vi "InitializeCamera.vi"() -> ()   [LabVIEW 2015]
uses:
  MVCAMSDK.dll
panel:
  in  "相机枚举":T1(ring)
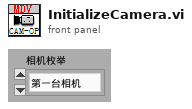
[diagram p1: front panel]
types:
  T1 = enum16{"第一台相机", "第二台相机", "第三台相机", "第四台相机", "第五台相机"}
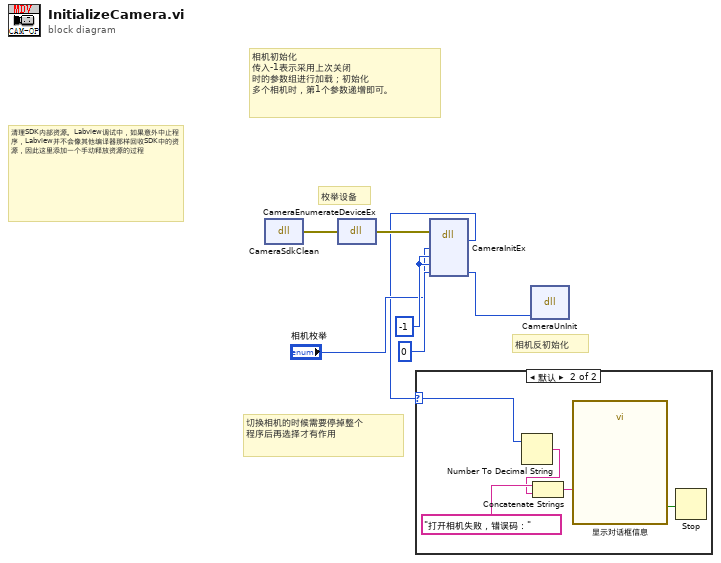
[diagram p0: block diagram]
diagram:
  w6 = -1
  # "相机反初始化"
  # "切换相机的时候需要停掉整个\n程序后再选择才有作用"
  # "清理SDK内部资源。Labview调试中，如果意外中止程序，Labview并不会像其他编译器那样回收SDK中的资源，因此这里添加一个手动释放资源的过程"
  # "相机初始化\n传入-1表示采用上次关闭\n时的参数组进行加载；初始化\n多个相机时，第1个参数递增即可。"
  # "枚举设备"
  n1 = dll-call lib="MVCAMSDK.dll" fn="CameraSdkClean"() -> (error out=w7:errorcluster)  [unwired: 4 in, 1 out]
  n2 = dll-call lib="MVCAMSDK.dll" fn="CameraEnumerateDeviceEx"(error in=w7) -> (error out=w4:errorcluster)  [unwired: 3 in, 1 out]
  n3 = dll-call lib="MVCAMSDK.dll" fn="CameraInitEx"(error in=w4, "相机索引值"="相机枚举", "参数加载方式"=w6, "要加载的参数组索引"=w6, "相机句柄"=0) -> ("返回类型"=w2:i32, "相机句柄"=w1:i32)  [unwired: 5 in, 2 out]
  n4 = case shown="默认" w2 {
    selector: w2 -> [_ w11]
    frame 0 {
    }
    frame Default {
      n5 = Number To Decimal String(number=w11) -> (decimal integer string=w8:string)  [unwired: 1 in]
      n6 = Concatenate Strings("打开相机失败，错误码：" ("字符串"), w8) -> (w10:string)
      n7 = call "显示对话框信息"("Message"=w10) -> ("结束"=w12:bool)  [unwired: 9 in, 1 out]
      n8 = Stop(stop? (T)=w12) -> ()
    }
  }
  n9 = dll-call lib="MVCAMSDK.dll" fn="CameraUnInit"("相机句柄"=w1) -> ()  [unwired: 5 in, 2 out]
